vi "Revision Query.vi"(8 "error in (no error)":errorcluster, 11 "heater_parent in":refnum<class "heater_parent.lvclass">) -> (0 "error out":errorcluster, 2 "Instrument Driver Revision":string, 3 "heater_parent out":refnum<class "heater_parent.lvclass">)   [LabVIEW 2020, in "polar_bear_plus_drivers.lvlib" / "heater_parent.lvclass"]
doc: "Queries the current instrument firmware revision and instrument driver revision.\n\nRefer to the Readme file for detailed driver information including modification history."
uses:
  <instrlib>/RxnRover/Driver Polar Bear Plus/heater_parent/heater_parent.lvclass
  <instrlib>/RxnRover/Driver Polar Bear Plus/polar_bear_plus_drivers.lvlib
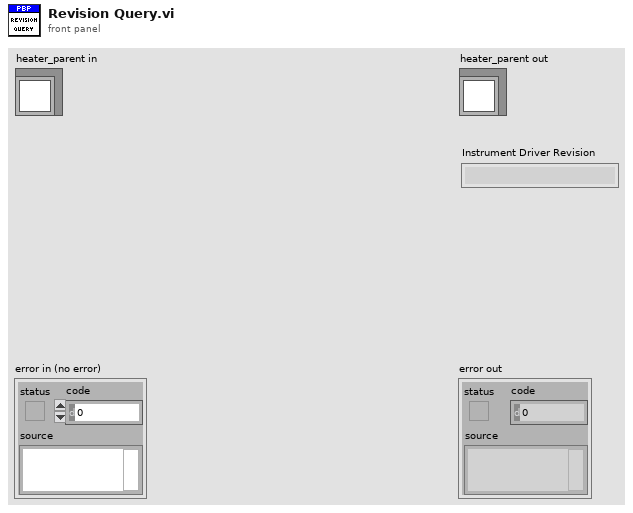
[diagram p1: front panel]
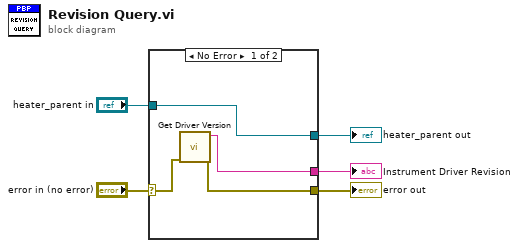
[diagram p0: block diagram]
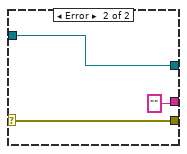
[diagram p2: hidden frame]
diagram:
  n1 = case shown="No Error" "error in (no error)" {
    selector: "error in (no error)" -> [w8 w12]
    tunnel: [w9 w12] -> w4
    tunnel: [w7 w11] -> w2
    tunnel: "heater_parent in" -> [w7 w11]
    tunnel: [w6 "" ("Instrument Driver Revision")] -> w1
    frame No Error {
      n2 = call <instrlib>:"Get Driver Version.vi"("error in (no error)"=w8) -> ("error out"=w9:errorcluster, "Instrument Driver Revision"=w6:string)  [unwired: 9 in]
    }
    frame Error {
    }
  }
  "error out" <- w4
  "heater_parent out" <- w2
  "Instrument Driver Revision" <- w1
